vi "SIM Get Nominated Time (reentrant).vi"(4 "simulation time":dbl, 5 "step size":dbl, 6 "proposed time":dbl, 7 "proposed step time":dbl) -> (3 "new proposed step time":dbl)   [LabVIEW 2017]
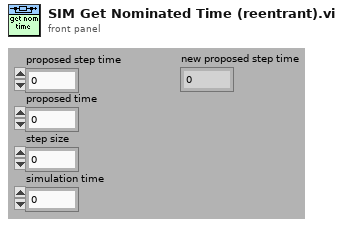
[diagram p1: front panel]
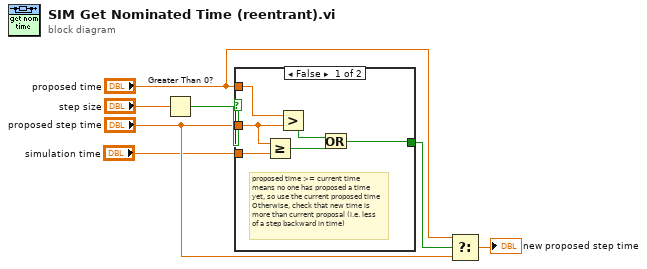
[diagram p0: block diagram]
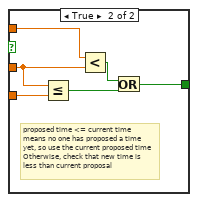
[diagram p2: hidden frame]
diagram:
  n1 = Greater Than 0?(x="step size") -> (x > 0?=w4:bool)
  n2 = case shown="False" w4 {
    tunnel: "proposed time" -> [w13 w19]
    tunnel: "proposed step time" -> [w9 w16]
    tunnel: [w12 w18] -> w7
    tunnel: "simulation time" -> [w10 w15]
    frame False {
      # "proposed time >= current time\nmeans no one has proposed a time\nyet, so use the current proposed time\nOtherwise, check that new time is\nmore than current proposal (i.e. less\nof a step backward in time)"
      n3 = Greater Or Equal?(x=w9, y=w10) -> (x >= y?=w8:bool)
      n4 = Greater?(x=w13, y=w9) -> (0:w11:bool)
      n5 = Or(x=w11, y=w8) -> (x .or. y?=w12:bool)
    }
    frame True {
      # "proposed time <= current time\nmeans no one has proposed a time\nyet, so use the current proposed time\nOtherwise, check that new time is\nless than current proposal"
      n6 = Less Or Equal?(x=w16, y=w15) -> (x <= y?=w14:bool)
      n7 = Less?(x=w19, y=w16) -> (x < y?=w17:bool)
      n8 = Or(x=w17, y=w14) -> (x .or. y?=w18:bool)
    }
  }
  n9 = Select(t="proposed time", s=w7, f="proposed step time") -> (s? t:f=→"new proposed step time":dbl)
